vi "String to Measurement Data.vi"() -> ()   [LabVIEW 2012]
panel:
  out "Measurement Data":T1
  out "Output":i32[](array[numeric])
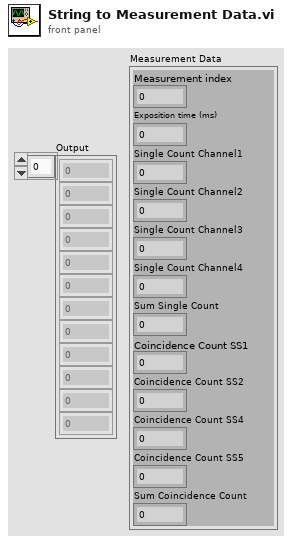
[diagram p1: front panel]
types:
  T1 = cluster{"Measurement index":i64, "Exposition time (ms)":i64, "Single Count Channel1":i64, "Single Count Channel2":i64, "Single Count Channel3":i64, "Single Count Channel4":i64, "Sum Single Count":i64, "Coincidence Count SS1":i64, "Coincidence Count SS2":i64, "Coincidence Count SS4":i64, "Coincidence Count SS5":i64, "Sum Coincidence Count":i64}
  T2 = cluster{"[0]":i64, "[1]":i64, "[2]":i64, "[3]":i64, "[4]":i64, "[5]":i64, "[6]":i64, "[7]":i64, "[8]":i64, "[9]":i64, "[10]":i64, "[11]":i64}
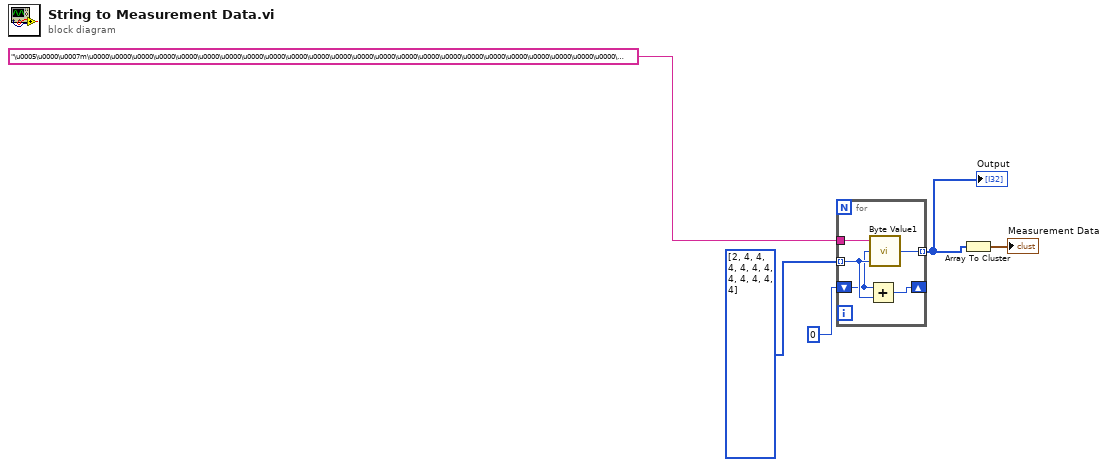
[diagram p0: block diagram]
diagram:
  n1 = for {
    tunnel: i8[] [2, 4, 4, 4, 4, 4, 4, 4, 4, 4, 4, 4] ("Length array") -> [w9] mode=indexing
    tunnel: "\u0005\u0000\u0007m\u0000\u0000\u0000\u0000\u0000\u0000\u0000\u0000\u0000\u0000\u0000\u0000\u0000\u0000\u0000\u0000\u0000\u0000\u0000\u0000\u0000\u0000\u0000\u0000\u0000\u0000\u0000\u0000\u0000\u0000\u0000\u0000\u0000\u0000\u0000\u0000\u0000\u0000\u0000\u0000\u0000\u0000" -> [w10]
    shift-right: [w8] -> _
    shift-left: i8 0 -> [w7]
    tunnel: [w6] -> w2 mode=indexing
    n2 = Add(x=w7, y=w9) -> (x+y=w8:i8)
    n3 = call "Byte Value1.vi"("Length"=w9, "Offset"=w7, "string"=w10) -> ("Value"=w6:i64)
  }
  "Output" <- w2
  n4 = Array To Cluster(array=w2) -> (cluster=→"Measurement Data":T2)
